vi "MGI Pad String.vi"(2 "Pad Character (\\s)":string=" ", 7 "String In":string, 13 "End Length":u32) -> (8 "String Out":string)   [LabVIEW 2020]
doc: "This VI adds as many pad characters as necessary to the end of <B>String In</B> to give it a length of <B>End Length</B>.\n\nAuthored by Robert C. Mortensen\nsupport@mooregoodideas.com\nwww.mooregoodideas.com\n\nCopyright (c) 2010, Moore Good Ideas, Inc.\n\nAll rights reserved.\n\nRedistribution and use in source and binary forms, with or without modification, are permitted provided that the following conditions are met:\n\n * Redistributions of source code must retain the above copyright notice, this list of conditions and the following disclaimer.\n * Redistributions in binary form must reproduce the above copyright notice, this list of conditions and the following disclaimer in the documentation and/or other materials provided with the distribution.\n * Neither the name of Moore Good Ideas, Inc. nor the names of its contributors may be used to endorse or promote products derived from this software without specific prior written permission.\n\nTHIS SOFTWARE IS PROVIDED BY THE COPYRIGHT HOLDERS AND CONTRIBUTORS \"AS IS\" AND ANY EXPRESS OR IMPLIED WARRANTIES, INCLUDING, BUT NOT LIMITED TO, THE IMPLIED WARRANTIES OF MERCHANTABILITY AND FITNESS FOR A PARTICULAR PURPOSE ARE DISCLAIMED. IN NO EVENT SHALL THE COPYRIGHT OWNER OR CONTRIBUTORS BE LIABLE FOR ANY DIRECT, INDIRECT, INCIDENTAL, SPECIAL, EXEMPLARY, OR CONSEQUENTIAL DAMAGES (INCLUDING, BUT NOT LIMITED TO, PROCUREMENT OF SUBSTITUTE GOODS OR SERVICES; LOSS OF USE, DATA, OR PROFITS; OR BUSINESS INTERRUPTION) HOWEVER CAUSED AND ON ANY THEORY OF LIABILITY, WHETHER IN CONTRACT, STRICT LIABILITY, OR TORT (INCLUDING NEGLIGENCE OR OTHERWISE) ARISING IN ANY WAY OUT OF THE USE OF THIS SOFTWARE, EVEN IF ADVISED OF THE POSSIBILITY OF SUCH DAMAGE."
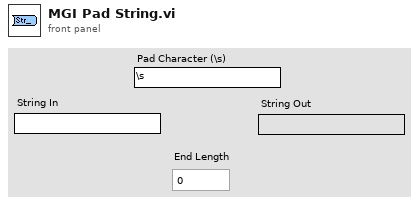
[diagram p1: front panel]
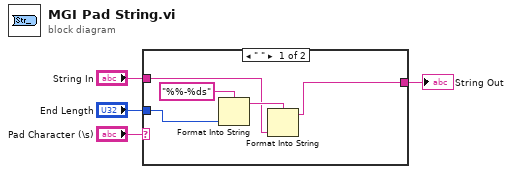
[diagram p0: block diagram]
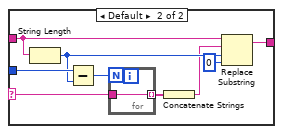
[diagram p2: hidden frame]
diagram:
  n1 = case shown="\" \"" "Pad Character (\\s)" {
    selector: "Pad Character (\\s)" -> [_ w10]
    tunnel: [w5 w18] -> w4
    tunnel: "String In" -> [w6 w17]
    tunnel: "End Length" -> [w8 w16]
    frame " " {
      n2 = Format Into String(format string="%%-%ds", w8) -> (resulting string=w7:string)  [unwired: 2 in, 1 out]
      n3 = Format Into String(format string=w7, w6) -> (resulting string=w5:string)  [unwired: 2 in, 1 out]
    }
    frame Default {
      n4 = String Length(string=w17) -> (length=w15:i32)
      n5 = Subtract(x=w16, y=w15) -> (x-y=w13:u32)
      n6 = for {
        N: w13 -> [_]
        tunnel: w10 -> [w19]
        tunnel: [w19] -> w12 mode=indexing
      }
      n7 = Concatenate Strings(w12) -> (w11:string)
      n8 = Replace Substring(2:0 ("length (len. of substring)"), 3:w15, 4:w11, 5:w17) -> (1:w18:string)  [unwired: 1 out]
    }
  }
  "String Out" <- w4
